vi "scan_unclick_stop_scan.vi"(8 "error in (no error)":errorcluster, 11 "scan_panel in":refnum<class "scan_panel.lvclass">) -> (0 "error out":errorcluster, 3 "scan_panel out":refnum<class "scan_panel.lvclass">)   [LabVIEW 2015, in "scan_panel.lvclass"]
uses:
  scan_panel.lvclass
  scan_panel.lvclass/scan_panel.ctl
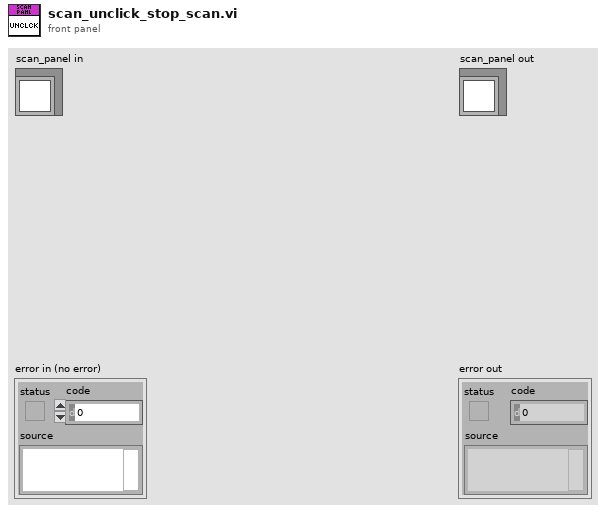
[diagram p1: front panel]
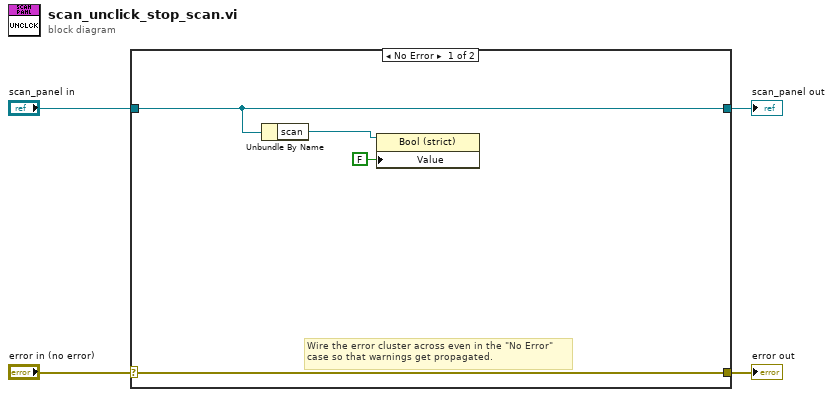
[diagram p0: block diagram]
diagram:
  n1 = case shown="No Error" "error in (no error)" {
    selector: "error in (no error)" -> [w8 w10]
    tunnel: [w8 w10] -> w3
    tunnel: [w7 w9] -> w1
    tunnel: "scan_panel in" -> [w7 w9]
    frame No Error {
      # "Wire the error cluster across even in the \"No Error\"\ncase so that warnings get propagated."
      n2 = Unbundle By Name(w7) -> ("scan"=w6:refnum<vi>)
      n3 = property class="Bool (strict)"(reference=w6, "Value"=FALSE) -> ()  [unwired: 1 in, 2 out]
    }
    frame Error {
    }
  }
  "error out" <- w3
  "scan_panel out" <- w1
